vi "SHUTTER_CCD.vi"(7 "Shutter State":u32, 8 "error out":errorcluster, 9 "Shutter Comp Time: Pre Open":u32, 10 "Shutter Comp Time: Post Open":u32, 11 "Camera Handle":u32) -> (0 "error out":errorcluster, 1 "String":string, 2 "INI Flag":bool, 3 "Camera Handle":u32)   [LabVIEW 2015]
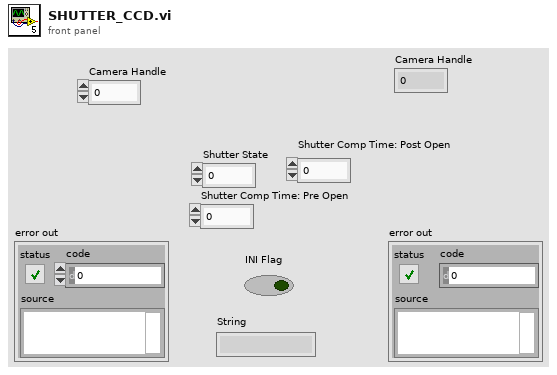
[diagram p1: front panel]
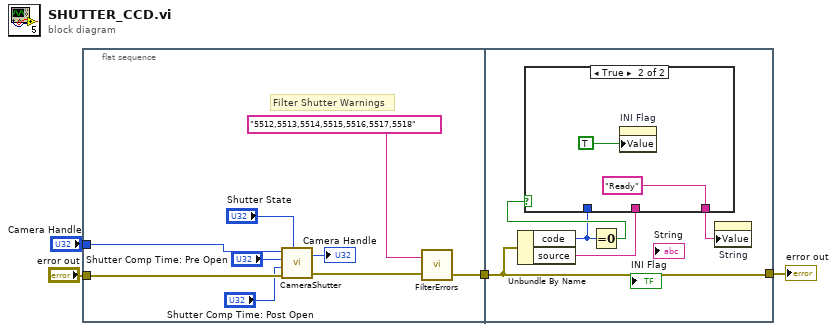
[diagram p0: block diagram]
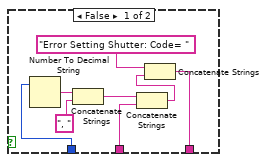
[diagram p2: hidden frame]
diagram:
  n1 = flat-sequence {
    tunnel: [w10] -> w4
    tunnel: "error out" -> [w12]
    tunnel: "Camera Handle" -> [w9]
    tunnel: w4 -> [w18]
    tunnel: [w18] -> w2
    frame #0 {
      # "Filter Shutter Warnings"
      n2 = call <userlib>:"CameraShutter.vi"("Camera Handle"=w9, "Shutter Comp Time: Pre Open"="Shutter Comp Time: Pre Open", "Shutter Comp Time: Post Open"="Shutter Comp Time: Post Open", "error in"=w12, "Shutter State"="Shutter State") -> ("Camera Handle"=→"Camera Handle":u32, "error out"=w11:errorcluster)
      n3 = call "FilterErrors.vi"("error in (no error)"=w11, "Error Numbers To Filter"="5512,5513,5514,5515,5516,5517,5518") -> ("error out"=w10:errorcluster)
    }
    frame #1 {
      n4 = Unbundle By Name(w18) -> ("code"=w15:i32, "source"=w16:string)
      n5 = Equal To 0?(x=w15) -> (x = 0?=w17:bool)
      n6 = case shown="True" w17 {
        tunnel: [w19 "Ready"] -> w14
        tunnel: w16 -> [w20 _]
        tunnel: w15 -> [w25 _]
        frame False {
          n7 = Number To Decimal String(number=w25) -> (decimal integer string=w24:string)  [unwired: 1 in]
          n8 = Concatenate Strings(w24, ", ") -> (w21:string)
          n9 = Concatenate Strings(w21, w20) -> (w22:string)
          n10 = Concatenate Strings("Error Setting Shutter: Code= ", w22) -> (w19:string)
        }
        frame True {
          n11 = property on="INI Flag" class="Bool (strict)"("Value"=TRUE) -> ()  [unwired: 2 in, 2 out]
        }
      }
      n12 = property on="String" class="Str"("Value"=w14) -> ()  [unwired: 2 in, 2 out]
    }
  }
  "error out" <- w2
